vi "close.vi"(8 "error in":errorcluster, 11 "E2E Tag Exchange runtime in":refnum<class "E2E Tag Exchange runtime.lvclass">) -> (0 "error out":errorcluster)   [LabVIEW 2017, in "E2E Tag Exchange runtime.lvclass"]
doc: "Provides an interface for terminating a module instance. While this interface performs no operations, a child should close and deallocate any open references or memory."
uses:
  E2E Tag Exchange runtime.lvclass
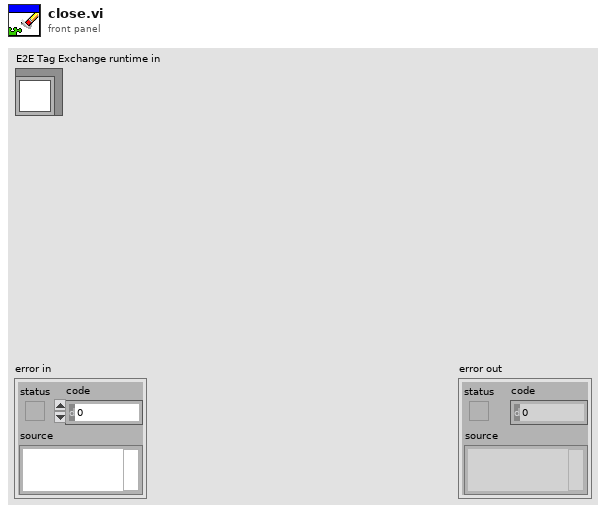
[diagram p1: front panel]
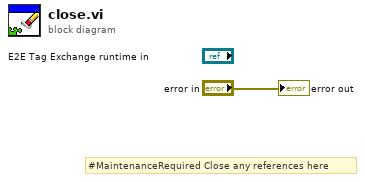
[diagram p0: block diagram]
diagram:
  # "#MaintenanceRequired Close any references here"
  "error out" <- "error in"
